vi "Serialize Properties.vi"(8 "error in (no error)":errorcluster, 10 "Properties":refnum<class "Property.lvclass">[](array[class]), 11 "Node in":refnum<k20>) -> (0 "error out":errorcluster, 3 "Node out":refnum<k20>)   [LabVIEW 2013, in "JUnit XML.lvlib" / "Test Suite.lvclass"]
uses:
  Test Suite.lvclass
  Property/Property.lvclass
  <vilib>/xml/Close Reference(Node).vi
  <vilib>/xml/NI_XML.lvlib
  JUnit XML.lvlib
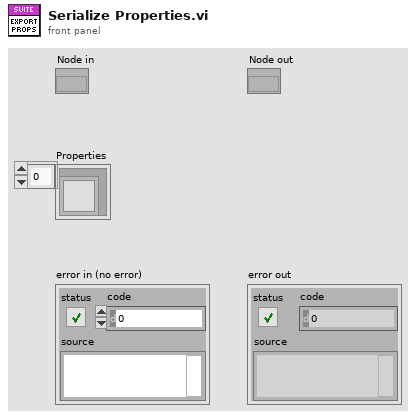
[diagram p1: front panel]
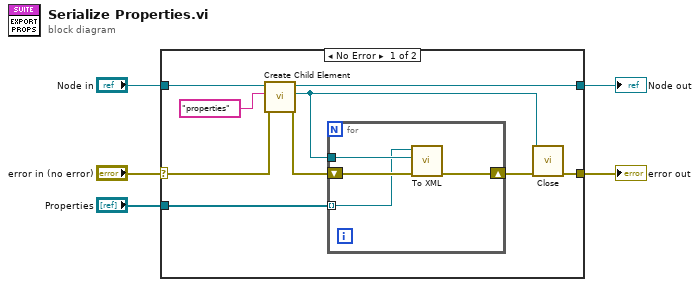
[diagram p0: block diagram]
diagram:
  n1 = case shown="No Error" "error in (no error)" {
    selector: "error in (no error)" -> [w7 w20]
    tunnel: "Node in" -> [w14 w19]
    tunnel: [w12 w20] -> w4
    tunnel: [w11 w19] -> w3
    tunnel: "Properties" -> [w9 _]
    frame No Error {
      n2 = call "Create Child Element.vi"("error in (no error)"=w7, "Name"="properties" ("Tag Name"), "Element in"=w14) -> ("error out"=w10:errorcluster, "Child Element"=w6:refnum<k20>, "Element out"=w11:refnum<k20>)  [unwired: 6 in]
      n3 = for {
        shift-right: [w17] -> w8
        shift-left: w10 -> [w16]
        tunnel: w9 -> [w15] mode=indexing
        tunnel: w6 -> [w18]
        n4 = call-dynamic "To XML.vi"("error in (no error)"=w16, "Parent"=w18, "Property in"=w15) -> ("error out"=w17:errorcluster)  [unwired: 8 in]
      }
      n5 = call-poly <vilib>:"Close.vi"("error in (no error)"=w8, "node"=w6) -> ("error out"=w12:errorcluster)  [unwired: 7 in]
    }
    frame Error {
    }
  }
  "error out" <- w4
  "Node out" <- w3
